vi "createNode.vi"(8 "error in (no error)":errorcluster, 10 "NodeSelection":T1, 11 "INodeFactory in":refnum<class "INodeFactory.lvclass">) -> (0 "error out":errorcluster, 2 "Node":refnum<class "Node.lvclass">, 3 "INodeFactory out":refnum<class "INodeFactory.lvclass">)   [LabVIEW 2016, in "INodeFactory.lvclass"]
uses:
  INodeFactory.lvclass
  Node/Node.lvclass
  Typedefs/NodeSelection.ctl
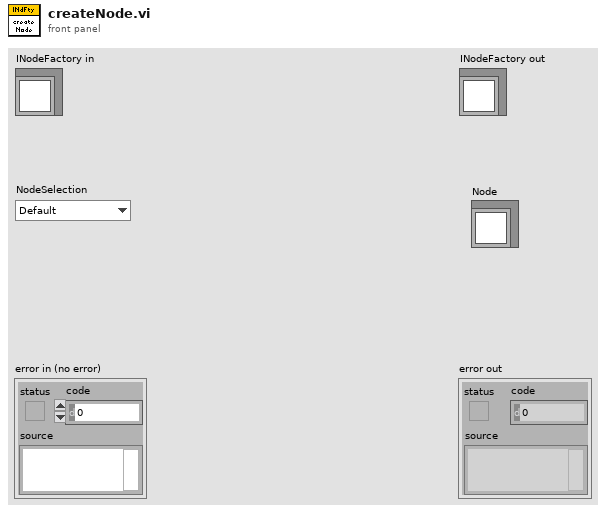
[diagram p1: front panel]
types:
  T1 = typedef "NodeSelection.ctl" = enum16{"Default", "CaseStructure", "EventStructure", "FlatSequence", "ForLoop", "WhileLoop"}
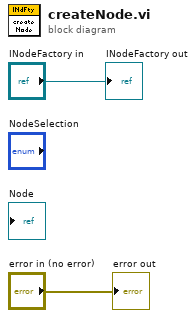
[diagram p0: block diagram]
diagram:
  "error out" <- "error in (no error)"
  "INodeFactory out" <- "INodeFactory in"
